vi "UIM Visibility Configuration.vi"() -> ()   [LabVIEW 2015]
doc: "This example shows that UIM can be used to organize different elements on the UI depending on what is needed at the moment. The user only needs to configure the specific amplitude and frequency so only the appropriate controls are made visible. This way the UI does not need to use tabs to organize elements."
uses:
  UIM/UIM.lvclass
  <vilib>/measure/NI_MABase.lvlib
panel:
  in  "Stop Button":bool
  in  "Square Frequency":dbl(knob)=2.350908061428739 scale=0.0..10.0
  in  "Square Amplitude":dbl(slide)=5.022026431718062 scale=0.0..10.0
  in  "Triangle Frequency":dbl(knob)=1.9305752303119406 scale=0.0..10.0
  in  "Triangle Amplitude":dbl(slide)=6.343612334801763 scale=0.0..10.0
  in  "Sine Frequency":dbl(knob)=1.2093081992493777 scale=0.0..10.0
  in  "Sine Amplitude":dbl(slide)=3.876651982378855 scale=0.0..10.0
  out "Waveform Graph":waveform(dbl)[](graph)=[{"t0"=timestamp(81.0 s since 1904-01-01), "dt"=0.001, "Y"=array[1000 elements]}, {"t0"=timestamp(81.0 s since 1904-01-01), "dt"=0.001, "Y"=array[1000 elements]}, {"t0"=timestamp(81.0 s since 1904-01-01), "dt"=0.001, "Y"=array[1000 elements]}]
  in  "Configuration":i32(listbox)
  # "Notice that these settings controls change"
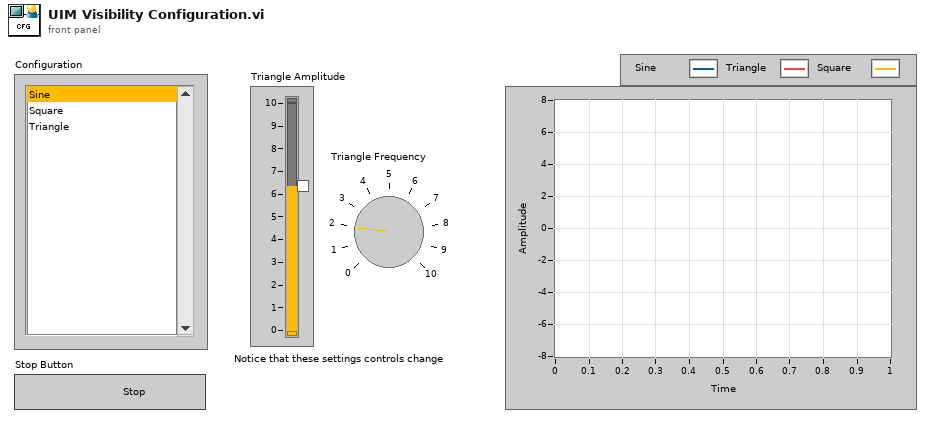
[diagram p1: front panel]
types:
  T1 = enum16{"Sine Wave", "Triangle Wave", "Square Wave", "Sawtooth Wave"}
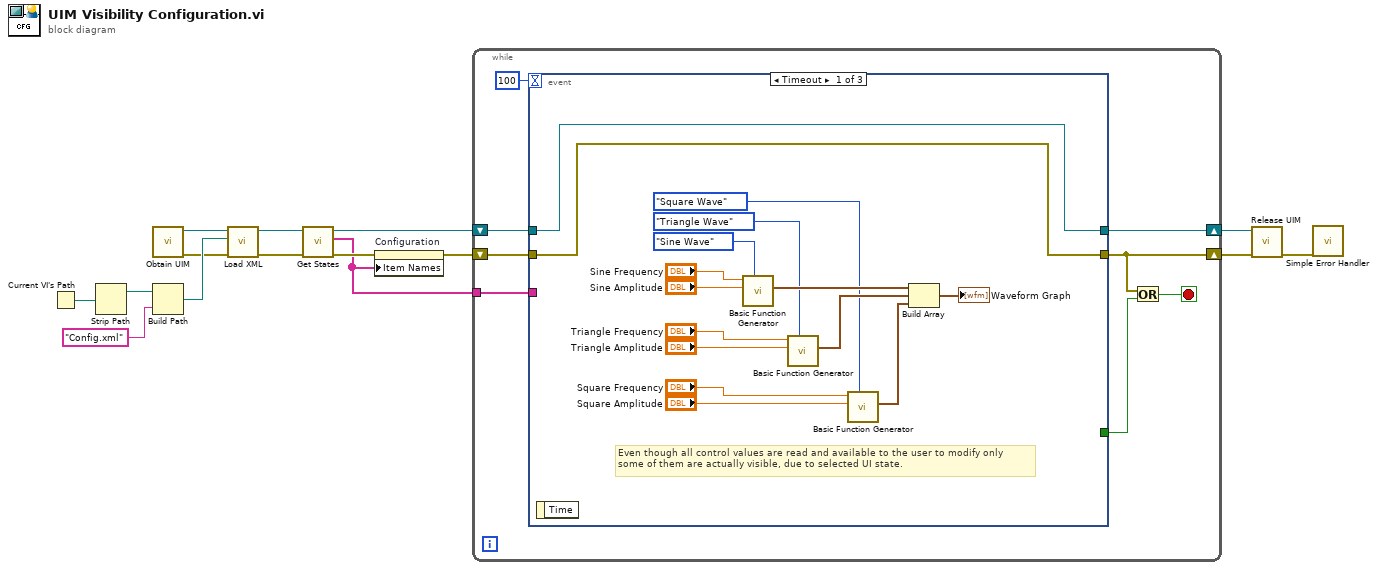
[diagram p0: block diagram]
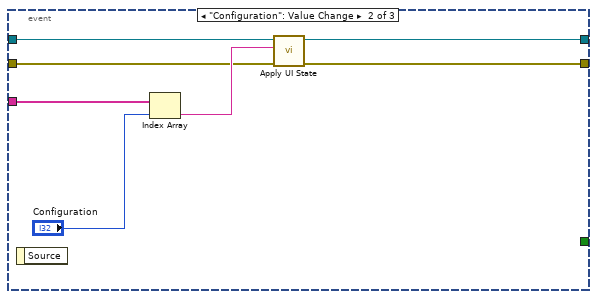
[diagram p2: hidden frame]
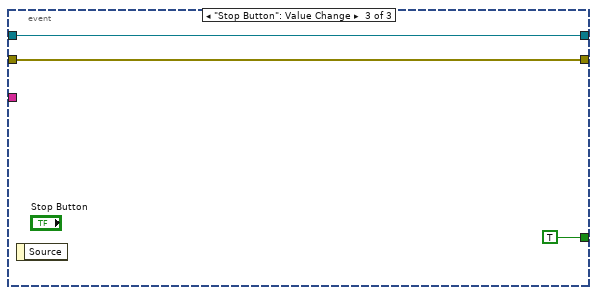
[diagram p3: hidden frame]
diagram:
  n1 = Current VI's Path() -> (path=w13:path)
  n2 = Strip Path(path=w13) -> (stripped path=w12:path)  [unwired: 1 out]
  n3 = call "Obtain UIM.vi"() -> ("Error Out"=w8:errorcluster, "UIM Handle"=w15:refnum<data-value>)  [unwired: 10 in]
  n4 = Build Path(base path=w12, name or relative path="Config.xml") -> (appended path=w11:path)
  n5 = call "Load XML.vi"("Error In"=w8, "XML File"=w11, "UIM In"=w15) -> ("Error Out"=w7:errorcluster, "UIM Out"=w10:refnum<data-value>)  [unwired: 7 in]
  n6 = call "Get States.vi"("Error In"=w7, "UIM In"=w10) -> ("Error Out"=w6:errorcluster, "States"=w4:string[], "UIM Out"=w9:refnum<data-value>)  [unwired: 7 in]
  n7 = property on="Configuration" class="LstBox (strict)"(error in=w6, "Item Names"=w4) -> (error out=w5:errorcluster)  [unwired: 1 in, 1 out]
  n8 = while {
    shift-right: [w16] -> w2
    shift-left: w5 -> [w21]
    shift-right: [w20] -> w3
    shift-left: w9 -> [w22]
    tunnel: w4 -> [w19]
    stop <- w17 stop-if-true
    n9 = event shown="[0] Timeout" {
      selector: _ -> [_ _ _]
      dyn-events: _ -> [_ _ _]
      timeout: 100 -> [_ _ _]
      tunnel: w22 -> [w24 w45 w48]
      tunnel: w21 -> [w25 w40 w47]
      tunnel: [w24 w44 w48] -> w20
      tunnel: w19 -> [_ w43 _]
      tunnel: [w25 w39 w47] -> w16
      tunnel: [_ _ TRUE] -> w18
      event Timeout {
        # "Even though all control values are read and available to the user to modify only\nsome of them are actually visible, due to selected UI state."
        n10 = event-data() -> ()  [unwired: 1 in, 1 out]
        n11 = call <vilib>:"Basic Function Generator.vi"("signal type"=T1."Sine Wave", "amplitude"="Sine Amplitude", "frequency"="Sine Frequency") -> ("signal out"=w29:waveform(dbl))  [unwired: 6 in, 2 out]
        n12 = call <vilib>:"Basic Function Generator.vi"("signal type"=T1."Triangle Wave", "amplitude"="Triangle Amplitude", "frequency"="Triangle Frequency") -> ("signal out"=w30:waveform(dbl))  [unwired: 6 in, 2 out]
        n13 = call <vilib>:"Basic Function Generator.vi"("signal type"=T1."Square Wave", "amplitude"="Square Amplitude", "frequency"="Square Frequency") -> ("signal out"=w31:waveform(dbl))  [unwired: 6 in, 2 out]
        n14 = Build Array(w29, w30, w31) -> (→"Waveform Graph":waveform(dbl)[])
      }
      event "Configuration": Value Change {
        n15 = event-data() -> ()  [unwired: 1 in, 1 out]
        n16 = Index Array(array=w43, index="Configuration") -> (element=w41:string)
        n17 = call "Apply UI State.vi"("Error In"=w40, "State Name"=w41, "UIM In"=w45) -> ("Error Out"=w39:errorcluster, "UIM Out"=w44:refnum<data-value>)  [unwired: 7 in]
      }
      event "Stop Button": Value Change {
        n18 = event-data() -> ()  [unwired: 1 in, 1 out]
      }
    }
    n19 = Or(x=w16, y=w18) -> (x .or. y?=w17:bool)
  }
  n20 = call "Release UIM.vi"("Error In"=w2, "UIM Handle"=w3) -> ("Error Out"=w1:errorcluster)  [unwired: 9 in]
  n21 = call <vilib>:"Simple Error Handler.vi"("error in (no error)"=w1) -> ()  [unwired: 4 in, 5 out]
